vi "multitone am.vi"() -> ()   [LabVIEW 2018]
uses:
  <vilib>/express/express analysis/Spectral/Block/exnSpectralBlock spectral measurements RMS poly.vi
  <vilib>/express/express analysis/Spectral/Block/exnSpectralBlock spectral measurements RMS DDT.vi
  <vilib>/express/express analysis/Spectral/XNode/ExpressSpectralMeasurementsBlockNode.xnode
panel:
  in  "Knob":dbl(knob) scale=0.0..1.0
  out "Waveform Graph 2":dynamicdata(graph)
  out "Waveform Graph":dynamicdata(graph)
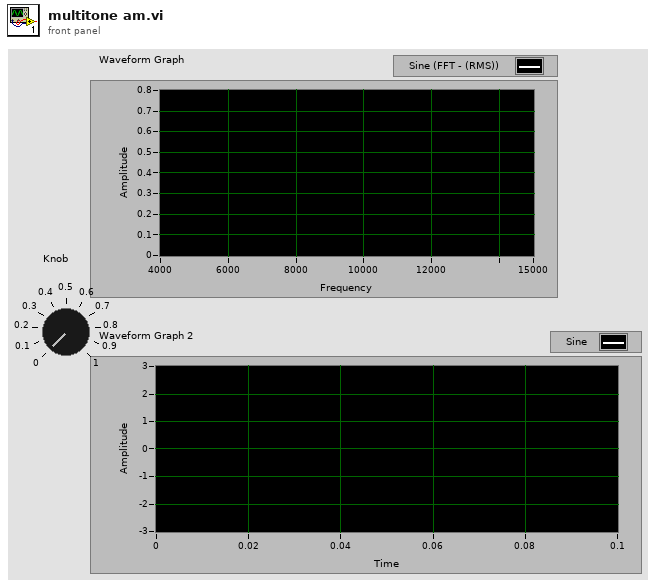
[diagram p1: front panel]
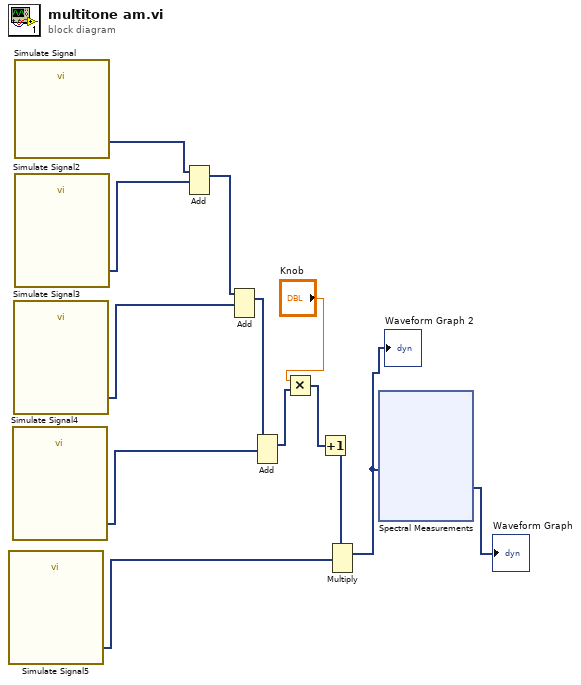
[diagram p0: block diagram]
diagram:
  n1 = call "Simulate Signal5"() -> ("Sine"=w7:dynamicdata)  [unwired: 14 in, 1 out]
  n2 = call "Simulate Signal4"() -> ("Sine"=w9:dynamicdata)  [unwired: 14 in, 1 out]
  n3 = call "Simulate Signal3"() -> ("Sine"=w11:dynamicdata)  [unwired: 14 in, 1 out]
  n4 = call "Simulate Signal"() -> ("Sine"=w13:dynamicdata)  [unwired: 14 in, 1 out]
  n5 = call "Simulate Signal2"() -> ("Sine"=w12:dynamicdata)  [unwired: 14 in, 1 out]
  n6 = Add(1:w12, 2:w13) -> (0:w10:dynamicdata)  [unwired: 1 in, 1 out]
  n7 = Add(1:w11, 2:w10) -> (0:w8:dynamicdata)  [unwired: 1 in, 1 out]
  n8 = Add(1:w9, 2:w8) -> (0:w2:dynamicdata)  [unwired: 1 in, 1 out]
  n9 = Multiply(x="Knob", y=w2) -> (x*y=w1:dynamicdata)
  n10 = Increment(x=w1) -> (x+1=w6:dynamicdata)
  n11 = Multiply(1:w7, 2:w6) -> (0:w4:dynamicdata)  [unwired: 1 in, 1 out]
  "Waveform Graph 2" <- w4
  n12 = xnode "Spectral Measurements"("Signals"=w4) -> ("FFT - (RMS)"=→"Waveform Graph":dynamicdata)  [unwired: 1 in, 2 out]
